vi "Actual Replot.vi"(8 "error in (no error)":errorcluster, 11 "MagLabGraph in":refnum<class "XY Plot.lvclass">) -> (0 "error out":errorcluster, 3 "MagLabGraph out":refnum<class "XY Plot.lvclass">)   [LabVIEW 2016, in "XY Plot.lvclass"]
uses:
  XY Plot.lvclass
  C:/github/LabActor/Plots/Plot/Plot.lvclass
  Plot/Plot.lvclass/Plot.ctl
  XY Plot.lvclass/XY Plot.ctl
  Plot/Read Data reduction.vi
  Plot/Plot.lvclass
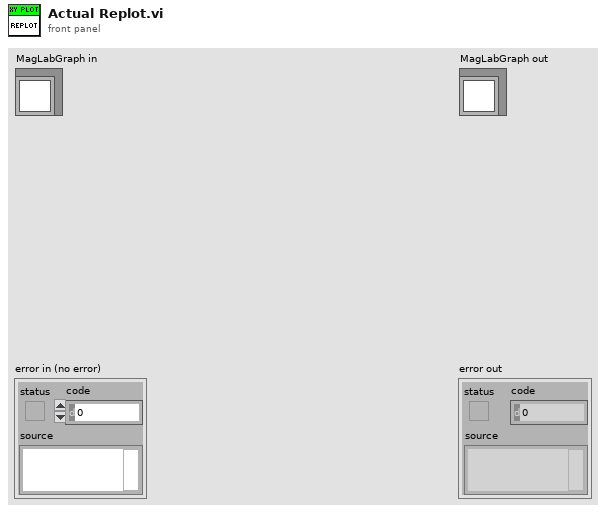
[diagram p1: front panel]
types:
  T1 = typedef "Data reduction.ctl" = cluster{"Clip time":bool, "Tiime 0":dbl, "Time 1":dbl, "Maximum data points":i32, "Decimation method":enum16{"coerce", "linear", "spline", "Min-Max", "Average"}}
  T2 = cluster{"File Path Control":path, "Group":string, "Channel":string, "Abbreviated":string}[]
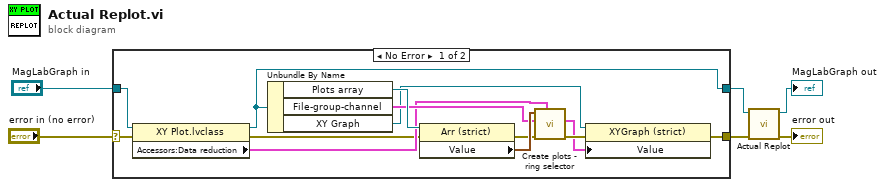
[diagram p0: block diagram]
diagram:
  n1 = case shown="No Error" "error in (no error)" {
    selector: "error in (no error)" -> [w7 w21]
    tunnel: [w14 w21] -> w4
    tunnel: [w10 w20] -> w2
    tunnel: "MagLabGraph in" -> [w19 w20]
    frame No Error {
      n2 = property class="XY Plot.lvclass"(reference=w19, error in=w7) -> (reference out=w10:refnum<class "XY Plot.lvclass">, error out=w8:errorcluster, "Accessors:Data reduction"=w9:T1)
      n3 = Unbundle By Name(w10) -> ("Plots array"=w18:refnum<vi>, "File-group-channel"=w16:T2, "XY Graph"=w13:refnum<vi>)
      n4 = property class="Arr (strict)"(reference=w18, error in=w8) -> (error out=w11:errorcluster, "Value"=w17:cluster{"X":u16, "Y":u16}[])  [unwired: 1 out]
      n5 = call "Create plots - ring selector.vi"("Data reduction"=w9, "Error In"=w11, "File-group-channel"=w16, "Plots  selector"=w17) -> ("Error Out"=w15:errorcluster, "Plots"=w12:cluster{dbl[], dbl[]}[])  [unwired: 6 in]
      n6 = property class="XYGraph (strict)"(reference=w13, error in=w15, "Value"=w12) -> (error out=w14:errorcluster)  [unwired: 1 out]
    }
    frame Error {
    }
  }
  n7 = call-parent "Actual Replot.vi"("error in (no error)"=w4, "Plot in"=w2) -> ("error out"=→"error out":errorcluster, "Plot out"=→"MagLabGraph out":refnum<class "XY Plot.lvclass">)  [unwired: 8 in]
